vi "Control Drive with Limelight.vi"(9 "X-DriveAuto":dbl, 11 "Y-DriveAuto":dbl) -> ()   [LabVIEW 2020]
uses:
  Framework/Robot Global Data.vi
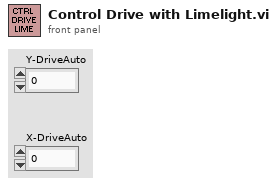
[diagram p1: front panel]
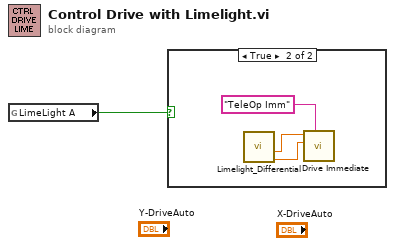
[diagram p0: block diagram]
diagram:
  n1 = global read "Robot Global Data.vi" "LimeLight A"() -> (w1:bool)
  n2 = case shown="True" w1 {
    frame False {
    }
    frame True {
      n3 = call "Limelight_Differential.vi"() -> ("DriveCommand"=w2:dbl, "SteerCommand"=w3:dbl)  [unwired: 8 in, 1 out]
      n4 = call "Drive Immediate.vi"("Description"="TeleOp Imm", "Right Setpoint"=w2, "Left Setpoint"=w3) -> ()  [unwired: 8 in, 1 out]
    }
  }
